vi "InitSnake.vi"(6 "Colors":T4={"HeadColor"=0, "BodyColor"=0, "TailColor"=0, "FeedColor"=16777224}, 7 "DisplaySize":T1, 8 "error in (no error)":errorcluster, 9 "HeadDirection":T2, 10 "HeadPos":T3, 11 "SnakeLength #BodyCells":u32) -> (0 "error out":errorcluster, 3 "Snake out":refnum<class "Snake.lvclass">)   [LabVIEW 2018, in "Snake.lvclass"]
uses:
  Snake.lvclass
  Typedefs/Colors.ctl
  Typedefs/XYposition.ctl
  Typedefs/UnitDirection.ctl
  Typedefs/DisplaySize.ctl
  Typedefs/CellType.ctl
  Snake.lvclass/Snake.ctl
  BodyCell/SnakeBodyCell.lvclass
panel:
  # "Connector Pane"
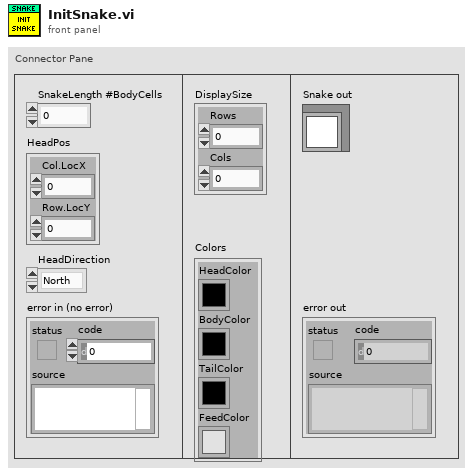
[diagram p1: front panel]
types:
  T1 = typedef "DisplaySize.ctl" = cluster{"Rows":i32, "Cols":i32}
  T2 = typedef "UnitDirection.ctl" = enum16{"North", "East", "South", "West"}
  T3 = typedef "XYposition.ctl" = cluster{"Col.LocX":i32, "Row.LocY":i32}
  T4 = typedef "Colors.ctl" = cluster{"HeadColor":u32, "BodyColor":u32, "TailColor":u32, "FeedColor":u32}
  T5 = typedef "CellType.ctl" = enum16{"Head", "Tail", "Body"}
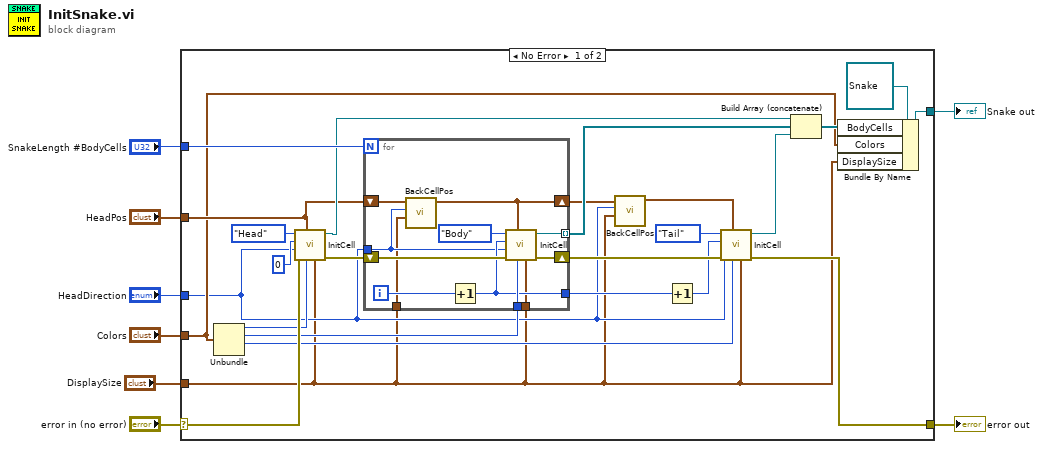
[diagram p0: block diagram]
diagram:
  n1 = case shown="No Error" "error in (no error)" {
    selector: "error in (no error)" -> [w30 w46]
    tunnel: [w27 w46] -> w7
    tunnel: [w32 _] -> w6
    tunnel: "SnakeLength #BodyCells" -> [w33 _]
    tunnel: "Colors" -> [w13 _]
    tunnel: "HeadDirection" -> [w10 _]
    tunnel: "HeadPos" -> [w15 _]
    tunnel: "DisplaySize" -> [w9 _]
    frame No Error {
      n2 = Unbundle(w13) -> ("HeadColor"=w25:u32, "BodyColor"=w24:u32, "TailColor"=w23:u32)  [unwired: 1 out]
      n3 = call "InitCell.vi"("DisplaySize"=w9, "Color"=w25, "HeadPos"=w15, "error in (no error)"=w30, "Direction"=w10, "CellPosInBody"=u16 0, "Cell"=CellType."Head") -> ("error out"=w31:errorcluster, "SnakeBodyCell out"=w18:refnum<class "SnakeBodyCell.lvclass">)  [unwired: 3 in]
      n4 = for {
        N: w33 -> [_]
        shift-right: [w44] -> w28
        shift-left: w31 -> [w45]
        tunnel: w24 -> [w42]
        tunnel: w10 -> [w38]
        tunnel: [w40] -> w21
        tunnel: [w39] -> w17 mode=indexing
        shift-right: [w36] -> w12
        shift-left: w15 -> [w37]
        tunnel: w9 -> [w35]
        tunnel: w9 -> [w34]
        i -> [w41]
        n5 = call "BackCellPos.vi"("DisplaySize"=w34, "Cell Direction"=w38, "Cell Pos"=w37) -> ("Back Cell Pos"=w36:T3)  [unwired: 8 in]
        n6 = Increment(x=w41) -> (x+1=w40:i32)
        n7 = call "InitCell.vi"("DisplaySize"=w35, "Color"=w42, "HeadPos"=w36, "error in (no error)"=w45, "Direction"=w38, "CellPosInBody"=w40, "Cell"=CellType."Body") -> ("error out"=w44:errorcluster, "SnakeBodyCell out"=w39:refnum<class "SnakeBodyCell.lvclass">)  [unwired: 3 in]
      }
      n8 = call "BackCellPos.vi"("DisplaySize"=w9, "Cell Direction"=w10, "Cell Pos"=w12) -> ("Back Cell Pos"=w11:T3)  [unwired: 8 in]
      n9 = Increment(x=w21) -> (x+1=w20:i32)
      n10 = call "InitCell.vi"("DisplaySize"=w9, "Color"=w23, "HeadPos"=w11, "error in (no error)"=w28, "Direction"=w10, "CellPosInBody"=w20, "Cell"=CellType."Tail") -> ("error out"=w27:errorcluster, "SnakeBodyCell out"=w16:refnum<class "SnakeBodyCell.lvclass">)  [unwired: 3 in]
      n11 = Build Array (concatenate)(w18, w17, w16) -> (w19:refnum<class "SnakeBodyCell.lvclass">[])
      n12 = Bundle By Name(cluster=refnum<class "Snake.lvclass"> refnum ("Snake in"), "BodyCells"=w19, "Colors"=w13, "DisplaySize"=w9) -> (w32:refnum<class "Snake.lvclass">)
    }
    frame Error {
    }
  }
  "error out" <- w7
  "Snake out" <- w6
